vi "Noise Reduction.vi"() -> ()   [LabVIEW 2023]
doc: "This example shows the application of the wavelet transforms in noise reduction.\n\nThe wavelet transform-based method can produce much higher denoising quality than conventional methods. The wavelet transform-based method can retain the details of a signal after denoising.\n\nThis example uses the WA Denoising VI to reduce noise in a simulated noisy signal.\n\n<b>Instructions:</b>\n1) Run this VI.\n2) Compare the <b>Noisy Signal</b> and the <b>Denoised Signal</b>.\n3) Double-click the Wavelet Denoise Express VI in the Block Diagram to change the denoising settings."
uses:
  <vilib>/Waveform/WDTOps.llb/WDT Number of Waveform Samples DBL.vi
  Instance           5 23Saved   Noise Reduction .vi
  <vilib>/addons/_Advanced Signal Processing/NI_AdvSigProcWA.lvlib
  <vilib>/measure/NI_MABase.lvlib
panel:
  in  "Data":u16(ring)=111 items=["1D Example Data"=100, "-"=101, "Doppler"=102, "HOP"=103, "TF Sine"=104, "Noisy Doppler"=105, "Sea Temperature"=106, "Sp500"=107, "Power Line"=108, "Engine Knocking"=109, "HeaviSine"=110, "Bumps"=111, "Blocks"=112, "Piece Regular"=113, "HypChirps"=114, "LinChirps"=115, "Chirps"=116, "Piece Polynomial"=117, "ECG"=131, "-"=118, "2D Example Data"=119, "-"=120, "Finger Print (Image)"=121, "Iris Flower (Image)"=122, "Mammogram (Image)"=123, "Lake (Image)"=127, "Two Can 1 (Image)"=132, "Two Can 2 (Image)"=133, "Camera Man (Image)"=134]
  in  "stop":bool
  out "Denoised Signal":waveform(dbl)(graph)
  out "Noisy Signal":waveform(dbl)(graph)
  # "Overview: Shows the application of the wavelet transforms in noise reduction.\nRequirements: LabVIEW Full Development System, Advanced Signal Processing Toolkit\nInstructions: \n1. Run this VI.\n2. Compare the Noisy Signal and the Denoised Signal.\n3. Double-click the Wavelet Denoise Express VI in the Block Diagram to change the denoising settings.\n4. Click Stop to stop the VI."
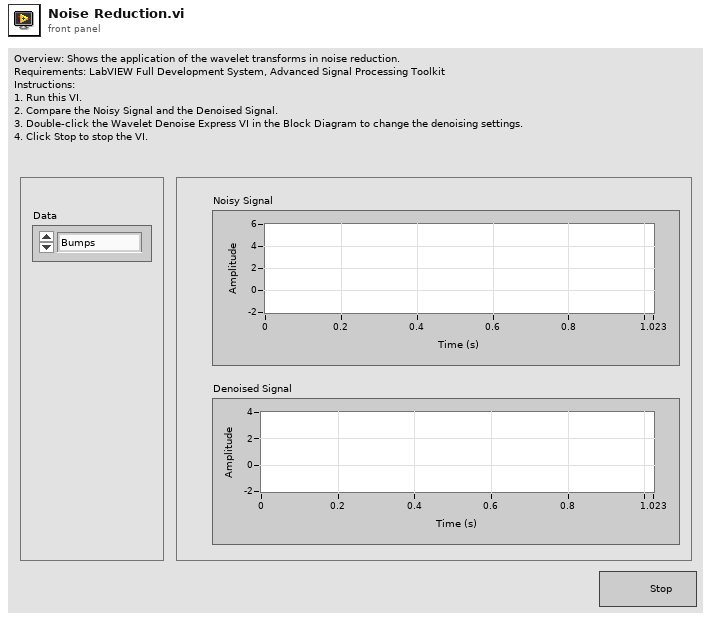
[diagram p1: front panel]
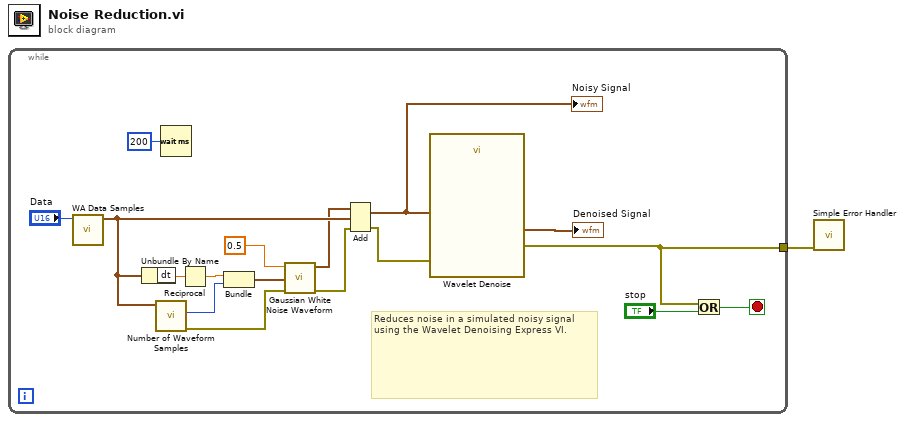
[diagram p0: block diagram]
diagram:
  n1 = while {
    tunnel: [w5] -> w1
    stop <- w7 stop-if-true
    # "Reduces noise in a simulated noisy signal using the Wavelet Denoising Express VI."
    n2 = call <vilib>:"WA Data Samples.vi"("data"="Data") -> ("signal"=w13:waveform(dbl))  [unwired: 10 out]
    n3 = Unbundle By Name(w13) -> ("dt"=w17:dbl)
    n4 = call-poly <vilib>:"Number of Waveform Samples.vi"("waveform in"=w13) -> ("error out"=w4:errorcluster, "number of samples"=w15:i32)  [unwired: 1 in, 8 out]
    n5 = Wait (ms)(milliseconds to wait=u32 200) -> ()  [unwired: 1 out]
    n6 = Reciprocal(x=w17) -> (1/x=w16:dbl)
    n7 = Bundle(w16, "number of samples"=w15) -> (w14:cluster{dbl, "number of samples":i32})  [unwired: 1 out]
    n8 = call <vilib>:"Gaussian White Noise Waveform.vi"("sampling info"=w14, "error in (no error)"=w4, "standard deviation"=0.5) -> ("error out"=w3:errorcluster, "signal out"=w12:waveform(dbl))  [unwired: 2 in, 5 out]
    n9 = Add(1:w13, 2:w12, 4:w3) -> (0:w9:waveform(dbl), 3:w2:errorcluster)
    "Noisy Signal" <- w9
    n10 = call "Wavelet Denoise"("error in (no error)"=w2, "Signal"=w9) -> ("error out"=w5:errorcluster, "Denoised Signal"=→"Denoised Signal":waveform(dbl))  [unwired: 8 out]
    n11 = Or(x=w5, y="stop") -> (x .or. y?=w7:bool)
  }
  n12 = call <vilib>:"Simple Error Handler.vi"("error in (no error)"=w1) -> ()  [unwired: 1 in, 8 out]
